vi "Configure External Trigger.vi"(4 "External Trigger Duration (1E-6)":dbl=1e-06 format="%^.2e", 5 "External Input Trigger Polarity (1: Negative)":u16(ring)=1 items=["Positive", "Negative"], 6 "External Trigger Delay (1E-5)":dbl=1e-05 format="%^.2e", 7 "External Output Trigger Polarity (0: Positive)":u16(ring) items=["Positive", "Negative"], 8 "error in (no error)":errorcluster, 9 "External Output Trigger Position (0: After)":u16(ring) items=["After", "Before"], 10 "External Output Trigger (F: Disable)":bool, 11 "VISA resource name":refnum<visa-resource-name>) -> (0 "error out":errorcluster, 3 "VISA resource name out":refnum<visa-resource-name>)   [LabVIEW 2018, in "Agilent ENA Series.lvlib"]
doc: "Configures external trigger.\n\nNotes:\n(1) TRIG:OUTP:DUR supported by E5063A and E5071C\n(2) TRIG:EXT:DEL not supported by E5061A, E5062A, E5072A, E5080A"
uses:
  Agilent ENA Series.lvlib
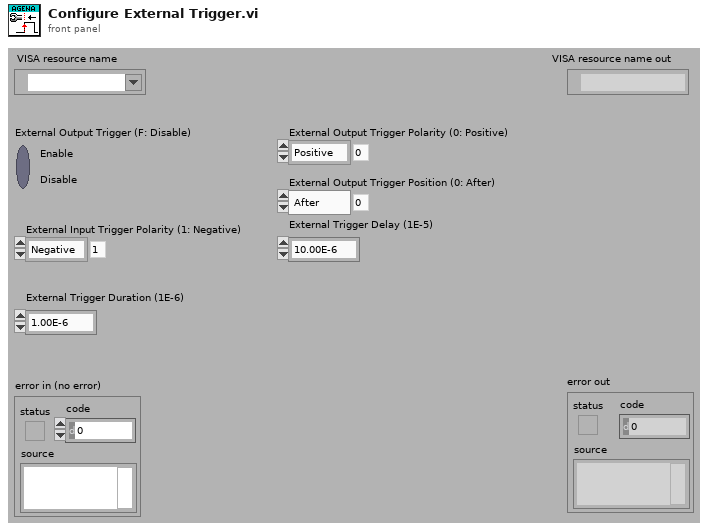
[diagram p1: front panel]
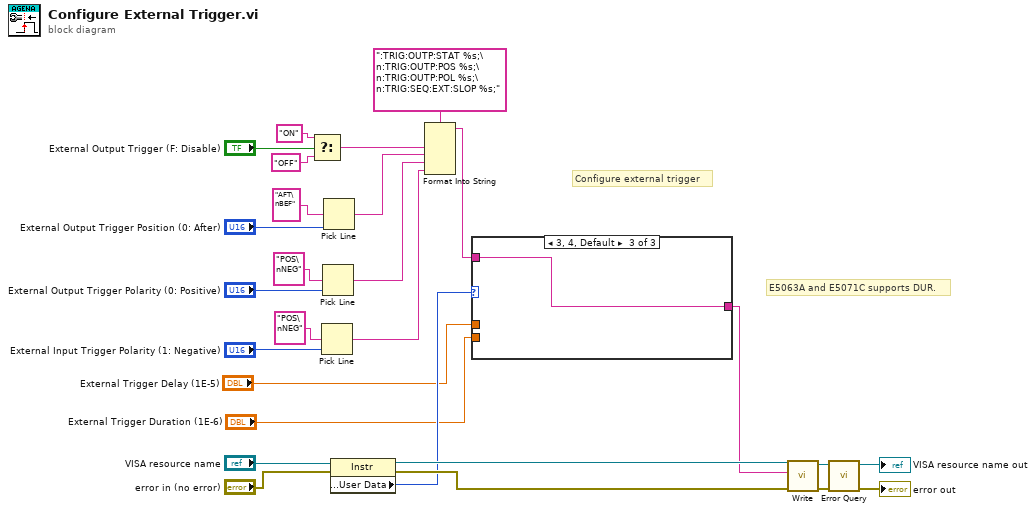
[diagram p0: block diagram]
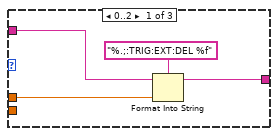
[diagram p2: hidden frame]
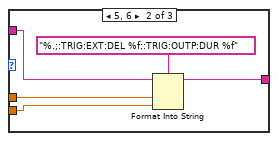
[diagram p3: hidden frame]
diagram:
  # "E5063A and E5071C supports DUR."
  # "Configure external trigger"
  n1 = Select(t="ON", s="External Output Trigger (F: Disable)", f="OFF") -> (s? t:f=w19:string)
  n2 = Pick Line(multi-line string="POS\nNEG", line index="External Input Trigger Polarity (1: Negative)") -> (output string=w10:string)  [unwired: 1 in]
  n3 = Pick Line(multi-line string="POS\nNEG", line index="External Output Trigger Polarity (0: Positive)") -> (output string=w14:string)  [unwired: 1 in]
  n4 = Pick Line(multi-line string="AFT\nBEF", line index="External Output Trigger Position (0: After)") -> (output string=w13:string)  [unwired: 1 in]
  n5 = property on="Property Node" class="Instr"(reference="VISA resource name", error in="error in (no error)") -> (reference out=w7:refnum<visa-resource-name>, error out=w6:errorcluster, "General Settings:User Data"=w5:u32)
  n6 = Format Into String(format string=":TRIG:OUTP:STAT %s;\n:TRIG:OUTP:POS %s;\n:TRIG:OUTP:POL %s;\n:TRIG:SEQ:EXT:SLOP %s;", w19, w13, w14, w10) -> (resulting string=w4:string)  [unwired: 2 in, 1 out]
  n7 = case shown="3, 4, Default" w5 {
    tunnel: w4 -> [w31 w36 w37]
    tunnel: "External Trigger Delay (1E-5)" -> [w30 w35 _]
    tunnel: [w28 w33 w37] -> w2
    tunnel: "External Trigger Duration (1E-6)" -> [_ w32 _]
    frame 0..2 {
      n8 = Format Into String(format string="%.;:TRIG:EXT:DEL %f", initial string=w31, w30) -> (resulting string=w28:string)  [unwired: 1 in, 1 out]
    }
    frame 5, 6 {
      n9 = Format Into String(format string="%.;:TRIG:EXT:DEL %f;:TRIG:OUTP:DUR %f", initial string=w36, w35, w32) -> (resulting string=w33:string)  [unwired: 1 in, 1 out]
    }
    frame 3, 4, Default {
    }
  }
  n10 = call "Write.vi"("error in (no error)"=w6, "String ()"=w2, "VISA resource name"=w7) -> ("error out"=w26:errorcluster, "VISA resource name out"=w27:refnum<visa-resource-name>)  [unwired: 6 in, 1 out]
  n11 = call "Error Query.vi"("error in (no error)"=w26, "VISA resource name"=w27) -> ("error out"=→"error out":errorcluster, "VISA resource name out"=→"VISA resource name out":refnum<visa-resource-name>)  [unwired: 6 in, 2 out]
